vi "Supply_ComplianceCheck.vi"(8 "error in (no error)":errorcluster, 11 "KE236 in":refnum<class "KE236.lvclass">) -> (0 "error out":errorcluster, 1 "Status string":string, 2 "Compliance exceeded?":bool, 3 "KE236 out":refnum<class "KE236.lvclass">)   [LabVIEW 2018, in "KE236.lvclass"]
uses:
  KE236.lvclass
  <vilib>/regexp/Match Regular Expression.xnode
  InstrControl.lvclass
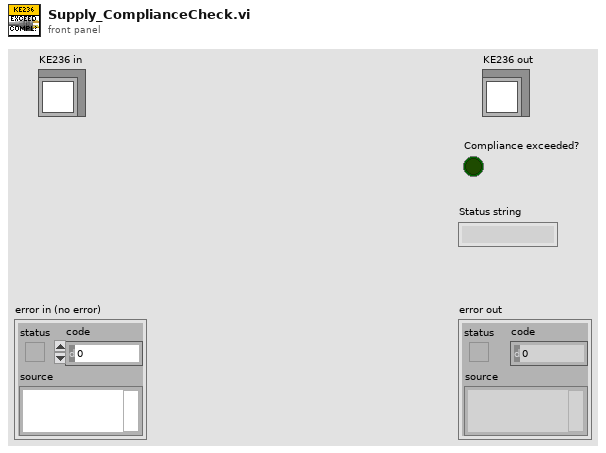
[diagram p1: front panel]
types:
  T1 = cluster{"error":bool, "code":i32, "source":string}
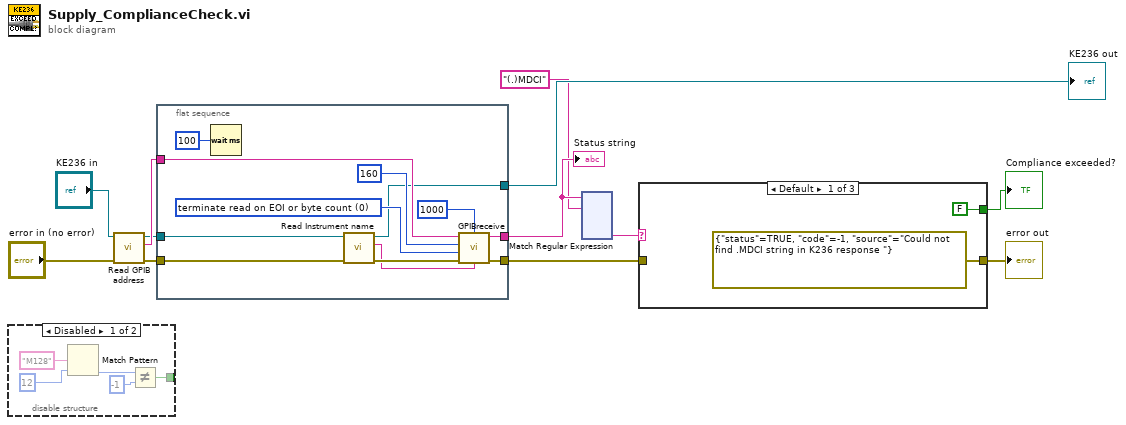
[diagram p0: block diagram]
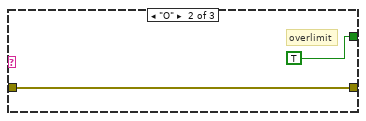
[diagram p2: hidden frame]
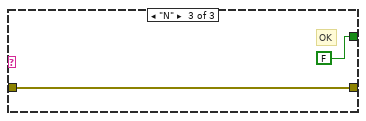
[diagram p3: hidden frame]
diagram:
  n1 = disable-structure shown="Disabled" {
    disable-tunnel: [w13 _] -> _
    frame Disabled {
      n2 = Match Pattern(regular expression="M128", offset (0)=12) -> (offset past match=w16:i32)  [unwired: 1 in, 3 out]
      n3 = Not Equal?(x=w16, y=-1) -> (x != y?=w13:bool)
    }
    frame Enabled {
    }
  }
  n4 = call-dynamic "Read GPIB address.vi"("error in (no error)"="error in (no error)", "InstControl in"="KE236 in") -> ("error out"=w9:errorcluster, "GPIB address"=w10:string, "InstControl out"=w8:refnum<class "KE236.lvclass">)  [unwired: 7 in]
  n5 = flat-sequence {
    tunnel: w10 -> [w29]
    tunnel: w9 -> [w21]
    tunnel: [w24] -> w6
    tunnel: [w23] -> w1
    tunnel: w8 -> [w22]
    tunnel: [w18] -> w7
    frame #0 {
      w26 = 0 items=["terminate read on EOI or byte count", "terminate read on EOI, byte count, or CR", "terminate read on EOI, byte count, or LF"] ("read mode")
      n6 = Wait (ms)(milliseconds to wait=u32 100) -> ()  [unwired: 1 out]
      n7 = call-dynamic "Read Instrument name.vi"("error in (no error)"=w21, "InstControl in"=w22) -> ("error out"=w20:errorcluster, "Instrument name"=w19:string, "InstControl out"=w18:refnum<class "KE236.lvclass">)  [unwired: 7 in]
      n8 = call "GPIBreceive.vi"("timeout ms"=u32 1000, "address string"=w29, "byte count"=160, "source"=w19, "read mode"=w26, "error in"=w20) -> ("read buffer"=w24:string, "error out"=w23:T1)  [unwired: 1 in, 1 out]
    }
  }
  n9 = xnode "Match Regular Expression"("input string"=w6, "regular expression"="(.)MDCI") -> ("submatch 1"=w4:string)  [unwired: 4 in, 5 out]
  n10 = case shown="Default" w4 {
    tunnel: [FALSE ("Compliance exceeded?") TRUE ("Compliance exceeded?") FALSE ("Compliance exceeded?")] -> w3
    tunnel: [errorcluster {"status"=TRUE, "code"=-1, "source"="Could not find .MDCI string in K236 response "} ("error out") w32 w34] -> w2
    tunnel: w1 -> [_ w32 w34]
    frame Default {
    }
    frame "O" {
      # "overlimit"
    }
    frame "N" {
      # "OK"
    }
  }
  "error out" <- w2
  "Compliance exceeded?" <- w3
  "KE236 out" <- w7
  "Status string" <- w6
